vi "Init Queues.vi"(8 "error in (no error)":errorcluster) -> (0 "error out":errorcluster)   [LabVIEW 2016, in "System.lvlib"]
uses:
  System.lvlib
  Controls/Control_Data Functions.ctl
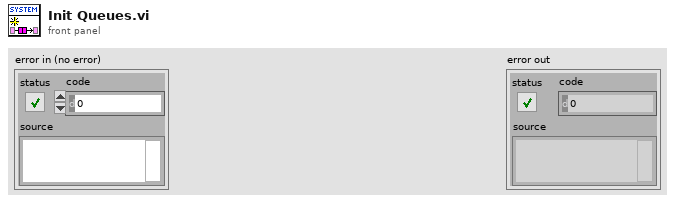
[diagram p1: front panel]
types:
  T1 = typedef "System.lvlib/Control_Data Functions.ctl" = enum16{"Get", "Set", "Release"}
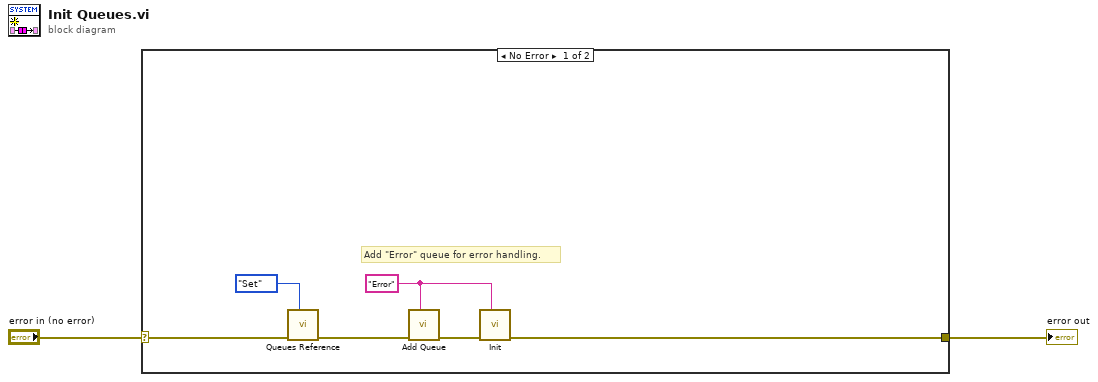
[diagram p0: block diagram]
diagram:
  n1 = case shown="No Error" "error in (no error)" {
    selector: "error in (no error)" -> [w8 w9]
    tunnel: [w3 w9] -> w1
    frame No Error {
      w4 = "Error" ("Process Name")
      # "Add \"Error\" queue for error handling."
      n2 = call "Queues Reference.vi"("Data Functions"=Control_Data_Functions."Set", "error in (no error)"=w8) -> ("error out"=w6:errorcluster)  [unwired: 8 in, 1 out]
      n3 = call "Add Queue.vi"("Process Name"=w4, "error in (no error)"=w6) -> ("error out"=w5:errorcluster)  [unwired: 9 in]
      n4 = call "Init.vi"("Process Name"=w4, "error in (no error)"=w5) -> ("error out"=w3:errorcluster)  [unwired: 9 in]
    }
    frame Error {
    }
  }
  "error out" <- w1
